vi "TEST - Get Physical Units from TD.vi"(8 "error in (no error)":errorcluster) -> (0 "error out":errorcluster, 2 "pass":bool)   [LabVIEW 2020]
uses:
  source/library/Type Descriptor.ctl
  source/library/Physical Units.ctl
panel:
  out "Failures":T3(array[cluster])
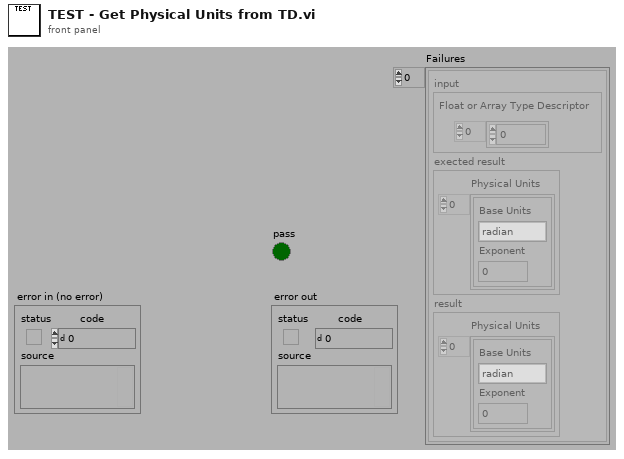
[diagram p1: front panel]
types:
  T1 = typedef "Type Descriptor.ctl" = i16[]
  T2 = typedef "Physical Units.ctl" = cluster{"Base Units":enum16{"radian", "steradian", "second", "meter", "kilogram", "ampere", "kelvin", "mole", "candela"}, "Exponent":i16}
  T3 = cluster{"input":cluster{"Float or Array Type Descriptor":T1}, "exected result":cluster{"Physical Units":T2[]}, "result":cluster{"Physical Units":T2[]}}[]
  T4 = cluster{"input":cluster{"Float or Array Type Descriptor":T1}, "exected result":cluster{"Physical Units":T2[]}, "result":cluster{"Physical Units":T2[]}}
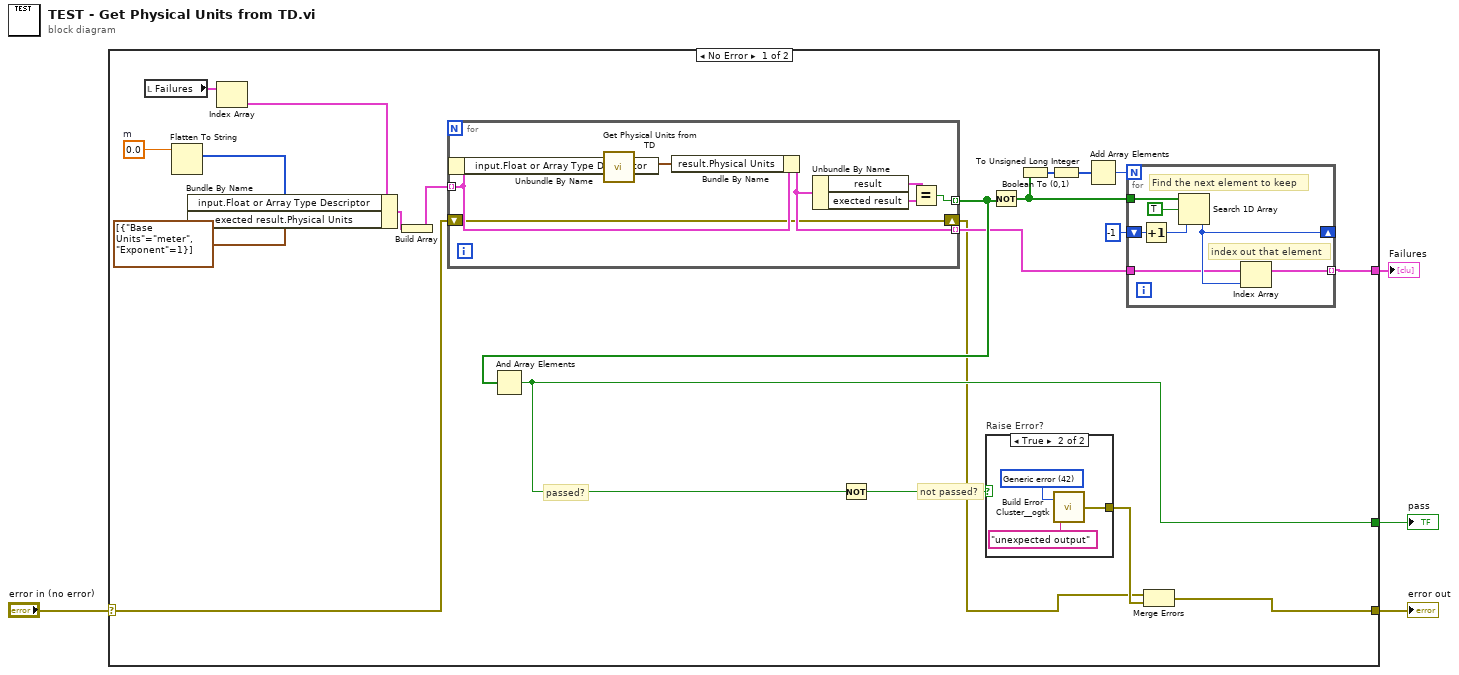
[diagram p0: block diagram]
diagram:
  n1 = case shown="No Error" "error in (no error)" {
    selector: "error in (no error)" -> [w11 w44]
    tunnel: [w22 _] -> w4
    tunnel: [w25 w44] -> w2
    tunnel: [w14 _] -> w1
    frame No Error {
      w7 = dbl[unit] 0.0  # m
      # "not passed?"
      # "passed?"
      n2 = local read "Failures"() -> (w9:T3)
      n3 = Flatten To String(anything=w7) -> (type string=w6:i16[])  [unwired: 3 in, 2 out]
      n4 = Index Array(array=w9) -> (element=w8:T4)  [unwired: 1 in]
      n5 = Bundle By Name(cluster=w8, "input.Float or Array Type Descriptor"=w6, "exected result.Physical Units"=T2[] [{"Base Units"=enum."meter", "Exponent"=1}] ("Physical Units")) -> (w13:T4)
      n6 = Build Array(w13) -> (w12:T3)
      n7 = for {
        tunnel: w12 -> [w39] mode=indexing
        tunnel: [w40] -> w16 mode=indexing
        tunnel: [w38] -> w15 mode=indexing
        shift-right: [w33] -> w10
        shift-left: w11 -> [w33]
        n8 = Unbundle By Name(w39) -> ("input.Float or Array Type Descriptor"=w35:T1)
        n9 = call "Get Physical Units from TD.vi"("Float or Array Type Descriptor"=w35) -> ("Physical Units"=w34:T2[])  [unwired: 9 in, 1 out]
        n10 = Bundle By Name(cluster=w39, "result.Physical Units"=w34) -> (w38:T4)
        n11 = Unbundle By Name(w38) -> ("result"=w37:cluster{"Physical Units":T2[]}, "exected result"=w36:cluster{"Physical Units":T2[]})
        n12 = Equal?(x=w37, y=w36) -> (x = y?=w40:bool)
      }
      n13 = And Array Elements(Boolean array=w16) -> (logical AND=w22:bool)
      n14 = Not(x=w22) -> (.not. x?=w23:bool)
      n15 = case "Raise Error?" shown="True" w23 {
        tunnel: [_ w41] -> w24
        frame False {
        }
        frame True {
          w42 = 42 items=["No error", "Argument error", "Memory is full", "Out of zone", "End of file", "File already open", "Generic file I/O error", "File not found", "File permission error", "Disk is full", "Duplicate path", "Too many files open", "System feature not enabled", "Resource file not found", "Cannot add resource", "Resource not found", "Image not found", "Image memory error", "Pen does not exist", "Config type invalid", "Config token not found", "Config parse error", "Config memory error", "Bad external code format", "Bad external code offset", "External code not present", "Null window", "Destroy window error", "Null menu", "Print aborted", "Bad print record", "Print driver error", "Windows error during printing", "Memory error during printing", "Print dialog error", "Generic print error", "Invalid device refnum", "Device not found", "Device parameter error", "Device unit error", "Cannot open device", "Device call aborted", "Generic error", "Cancelled by user", "Object ID too low", "Object ID too high", "Object not in heap", "Unknown heap", "Unknown object (invalid DefProc)", "Unknown object (DefProc not in table)", "Message out of range", "Invalid (null) method", "Unknown message", "Manager call not supported", "Bad address", "Network operation in progress", "Network operation timed out", "Connection is busy", "Network attribute not supported", "Network error", "Address in use", "System out of memory", "Connection aborted", "Connection refused", "Not connected", "Already connected", "Connection closed", "Initialization error (interapplication manager)", "Bad occurrence", "Wait on unbound occurrence handler", "Occurrence queue overflow", "Datalog type conflict", "Unused", "Unrecognized type (interapplication manager)", "Memory corrupt", "Failed to make temporary DLL", "Old CIN version", "Drag socket not found", "Failed to load drop-object", "Failed to register OLE object", "Failed to release OLE object", "Format specifier type mismatch", "Unknown format specifier", "Too few format specifiers", "Too many format specifiers", "Scan failed", "Newer CIN version", "Error converting to variant", "Runtime menu error", "Password tampered", "Variant attribute not found", "Incompatible variant data type", "Event data is not available", "Event Store is not present", "Occurrence is not found", "Event Queue is not created", "Event info is not available", "Refnum passed is NULL", "Error retrieving Class GUID", "Error retrieving CoClass GUID", "Error retrieving TypeLib GUID.", "Bad built application magic bytes.", "Specific driver is different from the specific driver associated with the Logical Name.", "There is no session opened to the class driver.", "Max Error", "MAX - Error with config objects", "MAX - Error loading configuration", "MAX - Group not supported"]
          n16 = call <userlib>:"Build Error Cluster__ogtk.vi"("String to Prepend to source (\"\")"="unexpected output" ("String to Prepend to source (\"\")"), "code"=w42) -> ("error out"=w41:errorcluster)
        }
      }
      n17 = Not(x=w16) -> (.not. x?=w18:bool[])
      n18 = Boolean To (0,1)(Boolean=w18) -> (0, 1=w19:i16[])
      n19 = To Unsigned Long Integer(number=w19) -> (unsigned 32bit integer=w17:u32[])
      n20 = Add Array Elements(numeric array=w17) -> (sum=w20:u32)
      n21 = for {
        N: w20 -> [_]
        tunnel: w15 -> [w28]
        tunnel: w18 -> [w32]
        shift-right: [w29] -> _
        shift-left: -1 ("start index (0)") -> [w30]
        tunnel: [w27] -> w14 mode=indexing
        # "index out that element"
        # "Find the next element to keep"
        n22 = Increment(x=w30) -> (x+1=w26:i32)
        n23 = Search 1D Array(1D array=w32, element=TRUE, start index (0)=w26) -> (index of element=w29:i32)
        n24 = Index Array(array=w28, index=w29) -> (element=w27:T4)
      }
      n25 = Merge Errors(w10, w24) -> (w25:errorcluster)
    }
    frame Error {
    }
  }
  "pass" <- w4
  "error out" <- w2
  "Failures" <- w1
